vi "TestStringSinkBufferMultipleOverflowAllEventsCaptured.vi"(8 "error in (no error)":errorcluster, 11 "TestCase in":refnum<class "TestStringControlSink.lvclass">) -> (0 "error out":errorcluster, 3 "TestCase out":refnum<class "TestStringControlSink.lvclass">)   [LabVIEW 2019, in "TestStringControlSink.lvclass"]
uses:
  TestStringControlSink.lvclass
  Source/String Formats/String Expression Format/String Expression Format.lvclass/String Expression Format.ctl
  Source/Composed Log/LoggerReference/LoggerReference.lvclass/LoggerReference.ctl
  7fc97478-71b4-4be4-9b40-44a1edbd2178.vi
  1ec4c22a-6b03-4cff-a1e2-0f91a771adcd.vi
  a54f4072-39c1-494a-b938-3c8b125e08bf.vi
  Source/String Formats/String Expression Format/Run Formatter.vi
  Source/Composed Log/LoggerReference/Return Aggregate Queues.vi
  Source/Composed Log/LoggerReference/Add Aggregate Log.vi
  7fc97478-71b4-4be4-9b40-44a1edbd2178.vi/af3b3336-f291-42a8-9b57-711866ed8ead.vi
  Source/Composed Log/LoggerReference/Log.vi
  Source/Composed Log/LoggerReference/Get Valid Event Time.vi
  <vilib>/dlg_ctls.llb/Space Constant.vi
  Source/Composed Log/LoggerReference/Send Add Sink.vi
  Source/Composed Log/LoggerReference/Remove Stale Logs.vi
  Source/String Formats/String Expression Format/String Expression Format.lvclass
  C:/CS/Log/Source/IStringFormat/IStringFormat.lvclass
  Source/String Control Sink/String Control Sink.lvclass
  C:/CS/Log/Source/Composed Log/Log Sink/Log Sink.lvclass
  Source/Composed Log/Application Logger/Launch Worker Loop.vi
  Source/Composed Log/LoggerReference/Initialize Logger Instance.vi
  Source/Composed Log/LoggerReference/LoggerReference.lvclass
  Source/Composed Log/IErrorFormat/IErrorFormat.lvclass
  Source/Composed Log/Log Sink/Log Sink.lvclass
  <vilib>/addons/_JKI Toolkits/VI Tester/TestCase.llb/TestCase.lvclass
  C:/Program Files (x86)/National Instruments/LabVIEW 2019/vi.lib/addons/_JKI Toolkits/VI Tester/TestCase.llb/TestCase.lvclass
panel:
  out "String":string
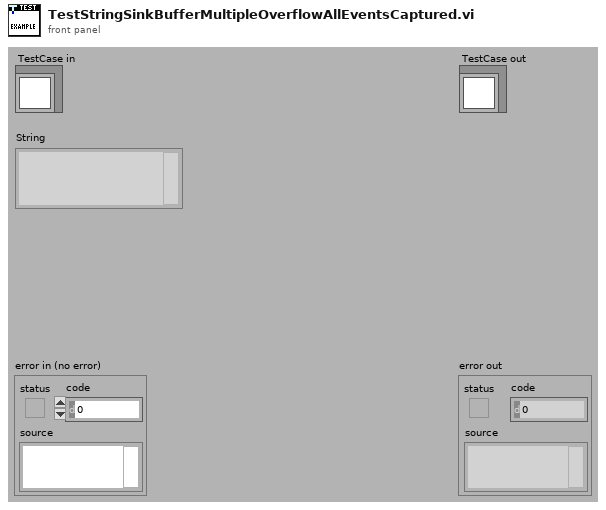
[diagram p1: front panel]
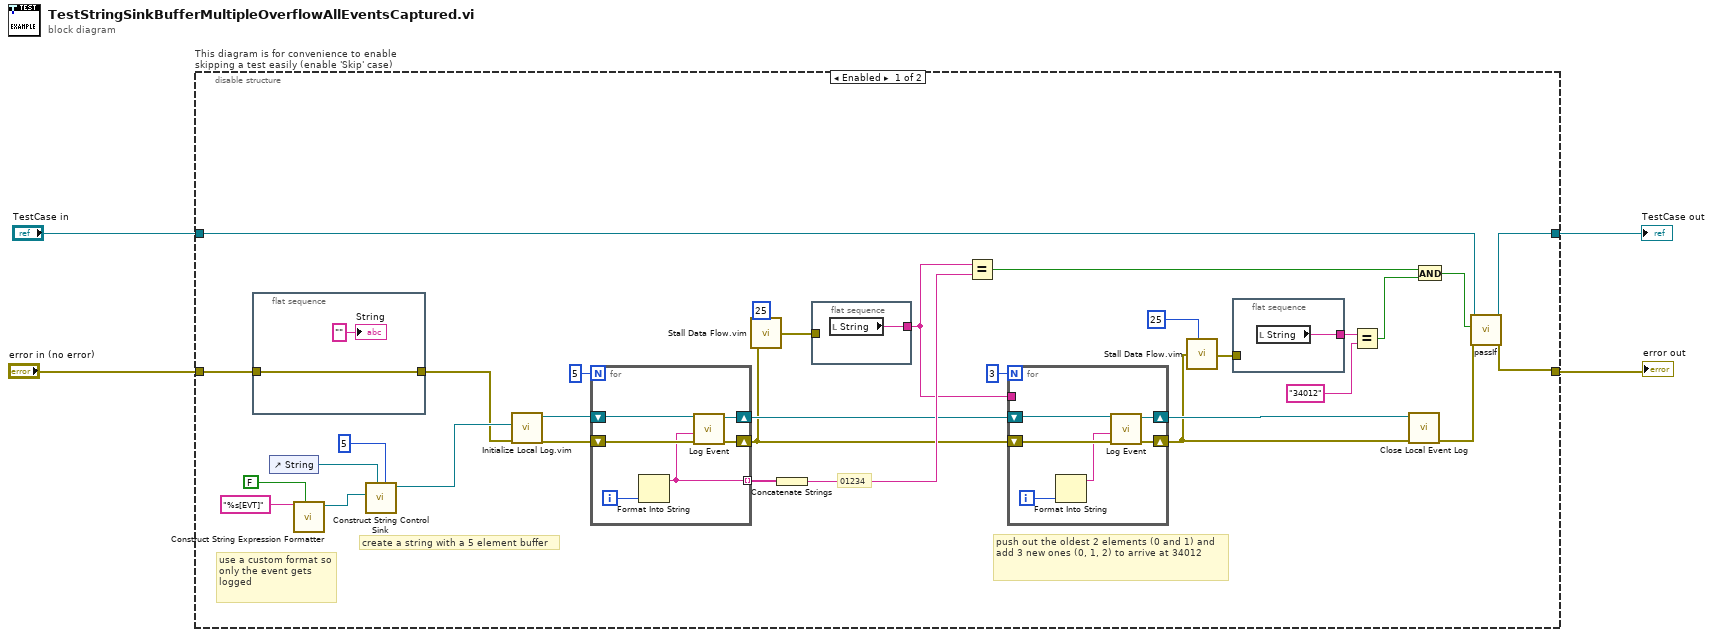
[diagram p0: block diagram]
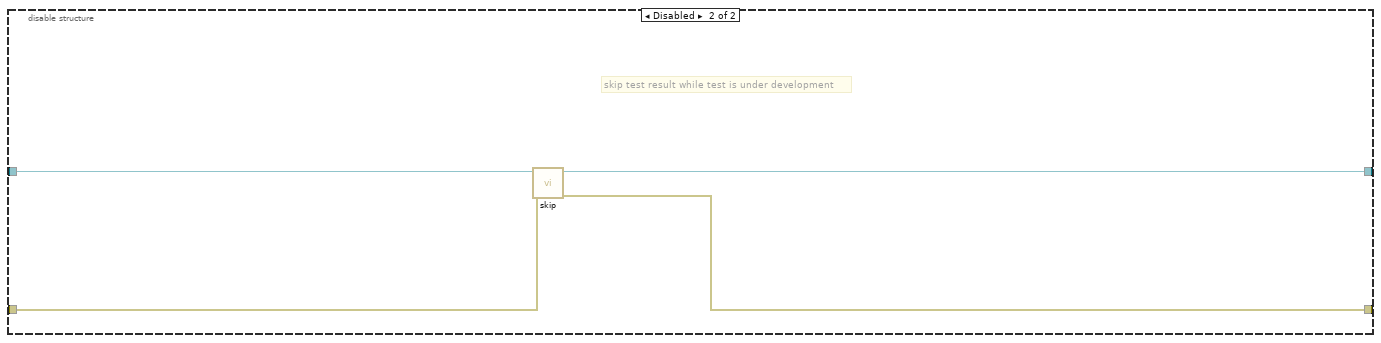
[diagram p2: hidden frame]
diagram:
  n1 = disable-structure "This diagram is for convenience to enable skipping a test easily (enable 'Skip' case)" shown="Enabled" {
    disable-tunnel: "TestCase in" -> [w36 w56]
    disable-tunnel: [w35 w54] -> w1
    disable-tunnel: [w34 w55] -> w3
    disable-tunnel: "error in (no error)" -> [w23 w53]
    frame Enabled {
      # "push out the oldest 2 elements (0 and 1) and add 3 new ones (0, 1, 2) to arrive at 34012"
      # "01234"
      # "create a string with a 5 element buffer"
      # "use a custom format so only the event gets logged"
      n2 = flat-sequence {
        tunnel: w23 -> [w45]
        tunnel: [w45] -> w22
        frame #0 {
          "String" <- "" ("String")
        }
      }
      n3 = control-ref of="String"() -> (w33:refnum<vi>)
      n4 = call "Construct String Expression Formatter.vi"("Append EOL?"=FALSE, "Format Specifier"="%s[EVT]") -> ("String Expression Format out"=w31:refnum<class "String Expression Format.lvclass">)  [unwired: 8 in, 1 out]
      n5 = call "Construct String Control Sink.vi"("Buffer Length(0)"=u32 5, "Str Refnum"=w33, "LogFormat"=w31) -> ("String Control Sink out"=w30:refnum<class "String Control Sink.lvclass">)  [unwired: 8 in]
      n6 = call "Initialize Local Log.vim"("error in (no error)"=w22, "Startup Sink(s)"=w30) -> ("error out"=w28:errorcluster, "Log Instance Reference"=w29:refnum<class "LoggerReference.lvclass">)  [unwired: 7 in, 1 out]
      n7 = for {
        N: 5 -> [_]
        shift-right: [w50] -> w17
        shift-left: w28 -> [w51]
        shift-right: [w48] -> w18
        shift-left: w29 -> [w52]
        tunnel: [w47] -> w20 mode=indexing
        i -> [w49]
        n8 = Format Into String(w49) -> (resulting string=w47:string)  [unwired: 3 in, 1 out]
        n9 = call "Log Event.vi"("error in (no error)"=w51, "Data To Log"=w47, "Log Instance"=w52) -> ("error out"=w50:errorcluster, "Log Instance Out"=w48:refnum<class "LoggerReference.lvclass">)  [unwired: 7 in]
      }
      n10 = call "Stall Data Flow.vim"("value in"=w17, "milliseconds to wait"=u32 25) -> ("value out"=w25:errorcluster)  [unwired: 1 out]
      n11 = Concatenate Strings(w20) -> (w19:string)
      n12 = flat-sequence {
        tunnel: [w46] -> w16
        tunnel: w25 -> [_]
        frame #0 {
          n13 = local read "String"() -> (w46:string)
        }
      }
      n14 = Equal?(x=w16, y=w19) -> (x = y?=w9:bool)
      n15 = for {
        N: 3 -> [_]
        shift-right: [w41] -> w14
        shift-left: w17 -> [w42]
        shift-right: [w39] -> w15
        shift-left: w18 -> [w43]
        tunnel: w16 -> [_]
        i -> [w40]
        n16 = Format Into String(w40) -> (resulting string=w38:string)  [unwired: 3 in, 1 out]
        n17 = call "Log Event.vi"("error in (no error)"=w42, "Data To Log"=w38, "Log Instance"=w43) -> ("error out"=w41:errorcluster, "Log Instance Out"=w39:refnum<class "LoggerReference.lvclass">)  [unwired: 7 in]
      }
      n18 = call "Stall Data Flow.vim"("value in"=w14, "milliseconds to wait"=u32 25) -> ("value out"=w13:errorcluster)  [unwired: 1 out]
      n19 = flat-sequence {
        tunnel: w13 -> [_]
        tunnel: [w37] -> w8
        frame #0 {
          n20 = local read "String"() -> (w37:string)
        }
      }
      n21 = Equal?(x=w8, y="34012") -> (x = y?=w7:bool)
      n22 = call "Close Local Event Log.vi"("error in (no error)"=w14, "Log Instance"=w15) -> ("error out"=w11:errorcluster)  [unwired: 9 in]
      n23 = And(x=w9, y=w7) -> (x .and. y?=w6:bool)
      n24 = call-dynamic "passIf.vi"("error in (no error)"=w11, "pass"=w6, "TestCase in"=w36) -> ("error out"=w34:errorcluster, "TestCase out"=w35:refnum<class "TestStringControlSink.lvclass">)  [unwired: 7 in]
    }
    frame Disabled {
      # "skip test result while test is under development"
      n25 = call <vilib>:"skip.vi"("error in (no error)"=w53, "TestCase in"=w56) -> ("error out"=w55:errorcluster, "TestCase out"=w54:refnum<class "TestStringControlSink.lvclass">)  [unwired: 8 in]
    }
  }
  "error out" <- w3
  "TestCase out" <- w1
